vi "has_GUI.vi"(8 "error in (no error)":errorcluster, 11 "GenericTraceProcessor in":refnum<class "GenericTraceProcessor.lvclass">) -> (0 "error out":errorcluster, 2 "has GUI?":bool, 3 "GenericTraceProcessor out":refnum<class "GenericTraceProcessor.lvclass">)   [LabVIEW 2010, in "GenericTraceProcessor.lvclass"]
uses:
  GenericTraceProcessor.lvclass
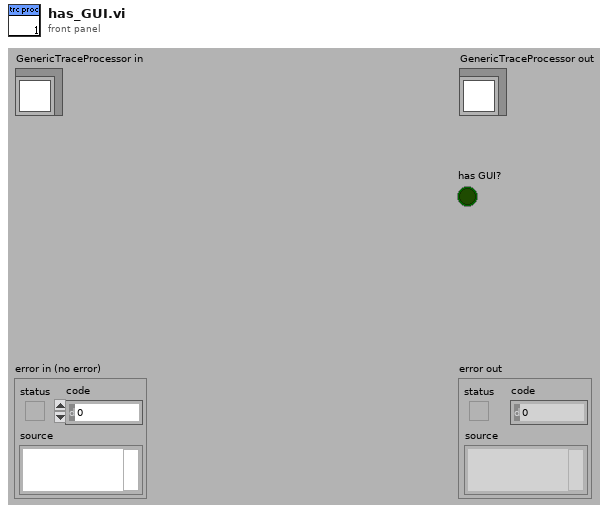
[diagram p1: front panel]
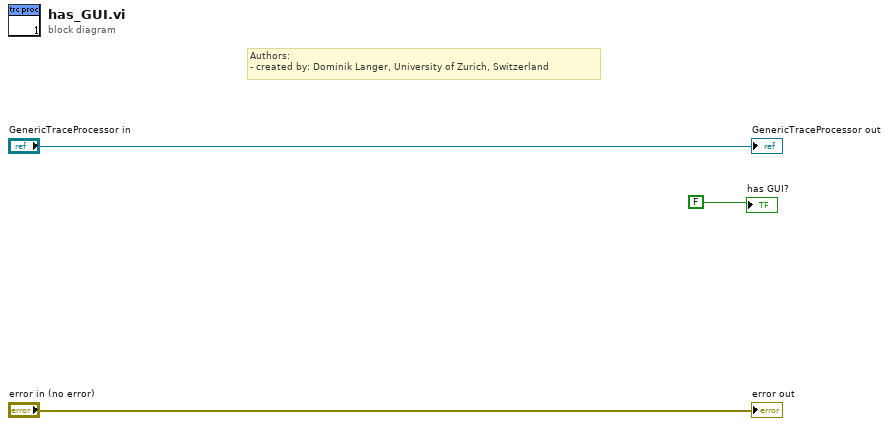
[diagram p0: block diagram]
diagram:
  # "Authors: \n- created by: Dominik Langer, University of Zurich, Switzerland"
  "error out" <- "error in (no error)"
  "GenericTraceProcessor out" <- "GenericTraceProcessor in"
  "has GUI?" <- FALSE
